vi "Simple Reader.vi"(8 "error in (no error)":errorcluster, 11 "CS580 Driver in":refnum<class "CS580 Driver.lvclass">) -> (0 "error out":errorcluster, 2 "Signals":dbl[](array[numeric]), 3 "CS580 Driver out":refnum<class "CS580 Driver.lvclass">)   [LabVIEW 2025, in "CS580 Driver.lvclass"]
uses:
  CS580 Driver.lvclass
  CS580 Driver.lvclass/CS580 Driver.ctl
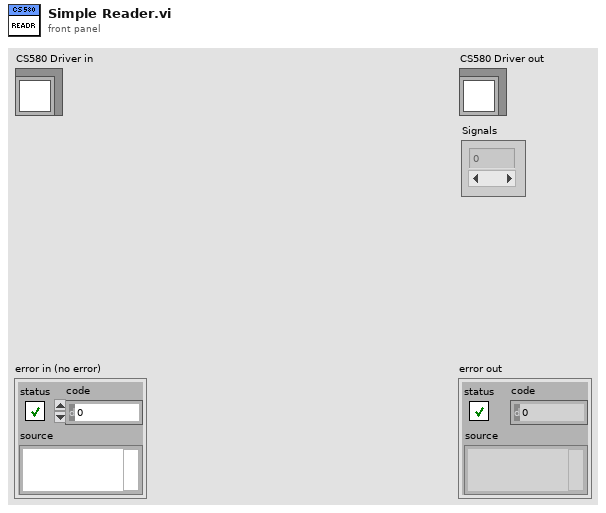
[diagram p1: front panel]
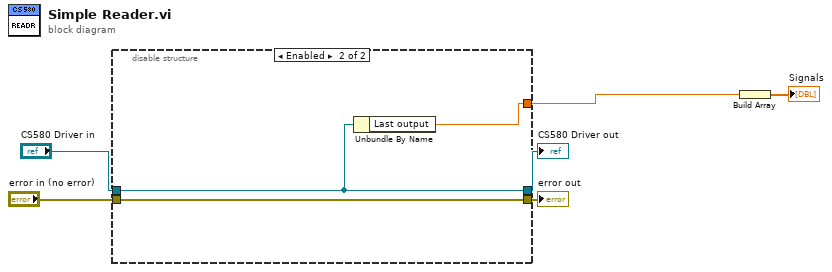
[diagram p0: block diagram]
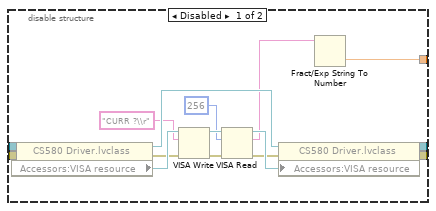
[diagram p2: hidden frame]
diagram:
  n1 = disable-structure shown="Enabled" {
    disable-tunnel: "CS580 Driver in" -> [w18 w23]
    disable-tunnel: "error in (no error)" -> [w17 w24]
    disable-tunnel: [w15 w24] -> w4
    disable-tunnel: [w14 w23] -> w3
    disable-tunnel: [w7 w22] -> w2
    frame Disabled {
      n2 = property class="CS580 Driver.lvclass"(reference=w18, error in=w17) -> (reference out=w21:refnum<class "CS580 Driver.lvclass">, error out=w19:errorcluster, "Accessors:VISA resource"=w20:refnum<visa-resource-name>)
      n3 = VISA Write(VISA resource name=w20, write buffer="CURR ?\\r" ("format string"), error in (no error)=w19) -> (VISA resource name out=w13:refnum<visa-resource-name>, error out=w10:errorcluster)  [unwired: 1 out]
      n4 = VISA Read(VISA resource name=w13, byte count=u32 256, error in (no error)=w10) -> (VISA resource name out=w12:refnum<visa-resource-name>, read buffer=w8:string, error out=w11:errorcluster)  [unwired: 1 out]
      n5 = property class="CS580 Driver.lvclass"(reference=w21, error in=w11, "Accessors:VISA resource"=w12) -> (reference out=w14:refnum<class "CS580 Driver.lvclass">, error out=w15:errorcluster)
      n6 = Fract/Exp String To Number(string=w8) -> (number=w7:dbl)  [unwired: 3 in, 1 out]
    }
    frame Enabled {
      n7 = Unbundle By Name(w23) -> ("Last output"=w22:dbl)
    }
  }
  "error out" <- w4
  "CS580 Driver out" <- w3
  n8 = Build Array(w2) -> (→"Signals":dbl[])
